vi "DamnYankeeFPGA.vi"() -> ()   [LabVIEW 2013]
doc: "This is the Damn Yankee FPGA code, at the moment it is only being used to read in the values from the remote control. We're using the FPGA to read a PWM signal because doing it in RT wasn't consistent enough.\n\nEric Schneider, May 2014"
uses:
  <vilib>/eio/EIONode/EIONode.xnode
  <vilib>/rvi/eio/common/nirviEmuTemplateMethod_errors.vi
panel:
  out "ConnectorA/DIO2":bool
  out "ConnectorA/DIO1":bool
  out "Sail ratio":sgl
  out "Rudder ratio":sgl
  out "Switch ratio":sgl
  out "Counter Out":i16
  out "High Counter Out":i16
  out "ConnectorA/DIO0":bool
  out "Counter In":i16
  out "High Counter In":i16
  out "Loop counter":i32
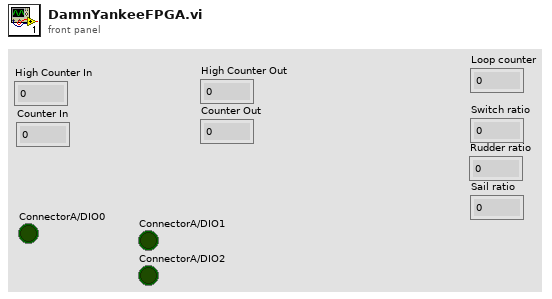
[diagram p1: front panel]
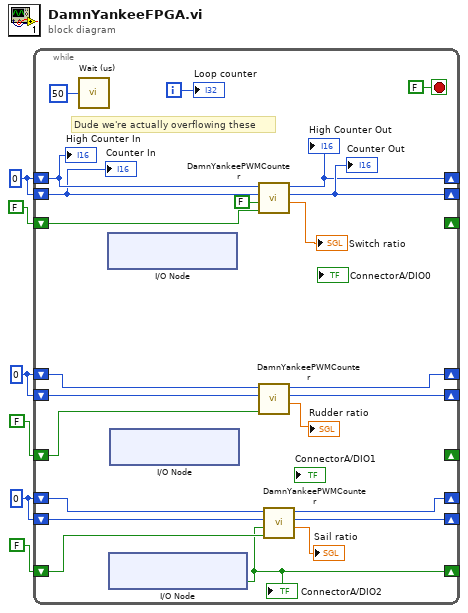
[diagram p0: block diagram]
diagram:
  w2 = i16 0 ("High Counter Out")
  w4 = i16 0 ("High Counter Out")
  w6 = i16 0 ("High Counter Out")
  n1 = while {
    shift-right: [w11] -> _
    shift-left: w6 -> [w29]
    shift-right: [w26] -> _
    shift-left: w6 -> [w28]
    shift-right: _ -> [_]
    shift-left: FALSE ("Jumped Up Out") -> [w27]
    shift-right: [w22] -> _
    shift-left: w4 -> [w21]
    shift-right: [w20] -> _
    shift-left: w4 -> [w19]
    shift-right: _ -> [_]
    shift-left: FALSE ("Jumped Up Out") -> [w18]
    shift-right: [w13] -> _
    shift-left: w2 -> [w14]
    shift-right: [w15] -> _
    shift-left: w2 -> [w16]
    shift-right: [w12] -> _
    shift-left: FALSE ("Jumped Up Out") -> [w17]
    i -> [w24]
    stop <- FALSE stop-if-true
    # "Dude we're actually overflowing these"
    n2 = call "Wait (us)"("Count(uSec)"=u32 50) -> ()  [unwired: 1 out]
    n3 = xnode "I/O Node"() -> ()  [unwired: 1 in, 2 out]
    n4 = xnode "I/O Node"() -> ("ConnectorA/DIO2"=w12:bool)  [unwired: 1 in, 1 out]
    "ConnectorA/DIO2" <- w12
    n5 = xnode "I/O Node"() -> ()  [unwired: 1 in, 2 out]
    n6 = call "DamnYankeePWMCounter.vi"("Old Value"=w27, "New Value"=FALSE, "Total Ticks In"=w28, "Ticks High In"=w29) -> ("Ratio"=→"Switch ratio":sgl, "Ticks Total Out"=w26:i16, "Ticks High Out"=w11:i16)  [unwired: 5 in]
    "High Counter Out" <- w11
    "Counter Out" <- w26
    n7 = call "DamnYankeePWMCounter.vi"("Old Value"=w18, "Total Ticks In"=w19, "Ticks High In"=w21) -> ("Ratio"=→"Rudder ratio":sgl, "Ticks Total Out"=w20:i16, "Ticks High Out"=w22:i16)  [unwired: 6 in]
    n8 = call "DamnYankeePWMCounter.vi"("Old Value"=w17, "New Value"=w12, "Total Ticks In"=w16, "Ticks High In"=w14) -> ("Ratio"=→"Sail ratio":sgl, "Ticks Total Out"=w15:i16, "Ticks High Out"=w13:i16)  [unwired: 5 in]
    "Loop counter" <- w24
    "High Counter In" <- w29
    "Counter In" <- w28
  }
